vi "slowcont.vi"() -> ()   [LabVIEW 2012]
uses:
  <vilib>/Instr/_visa.llb/VISA Configure Serial Port (Instr).vi
panel:
  out "total magnetic field":dbl(graph)
  out "magnetic field z coordinate":dbl(graph)
  out "magnetic field y coordinate":dbl(graph)
  out "magnetic field x coordinate":dbl(graph)
  out "Pressure":dbl(graph)
  out "humidity":dbl(graph)
  out "Temperature":dbl(graph)
  out "array type (2D Dbl) 2":string[](array[string])
  out "array type (2D Dbl)":string[](array[string])
  out "array 2":string[](array[string])
  out "read buffer":string
  in  "stop":bool
  in  "VISA resource name":refnum<visa-resource-name>="COM5"
  in  "XOFF Character":u8=19 format="%.0x"
  in  "XON Character":u8=17 format="%.0x"
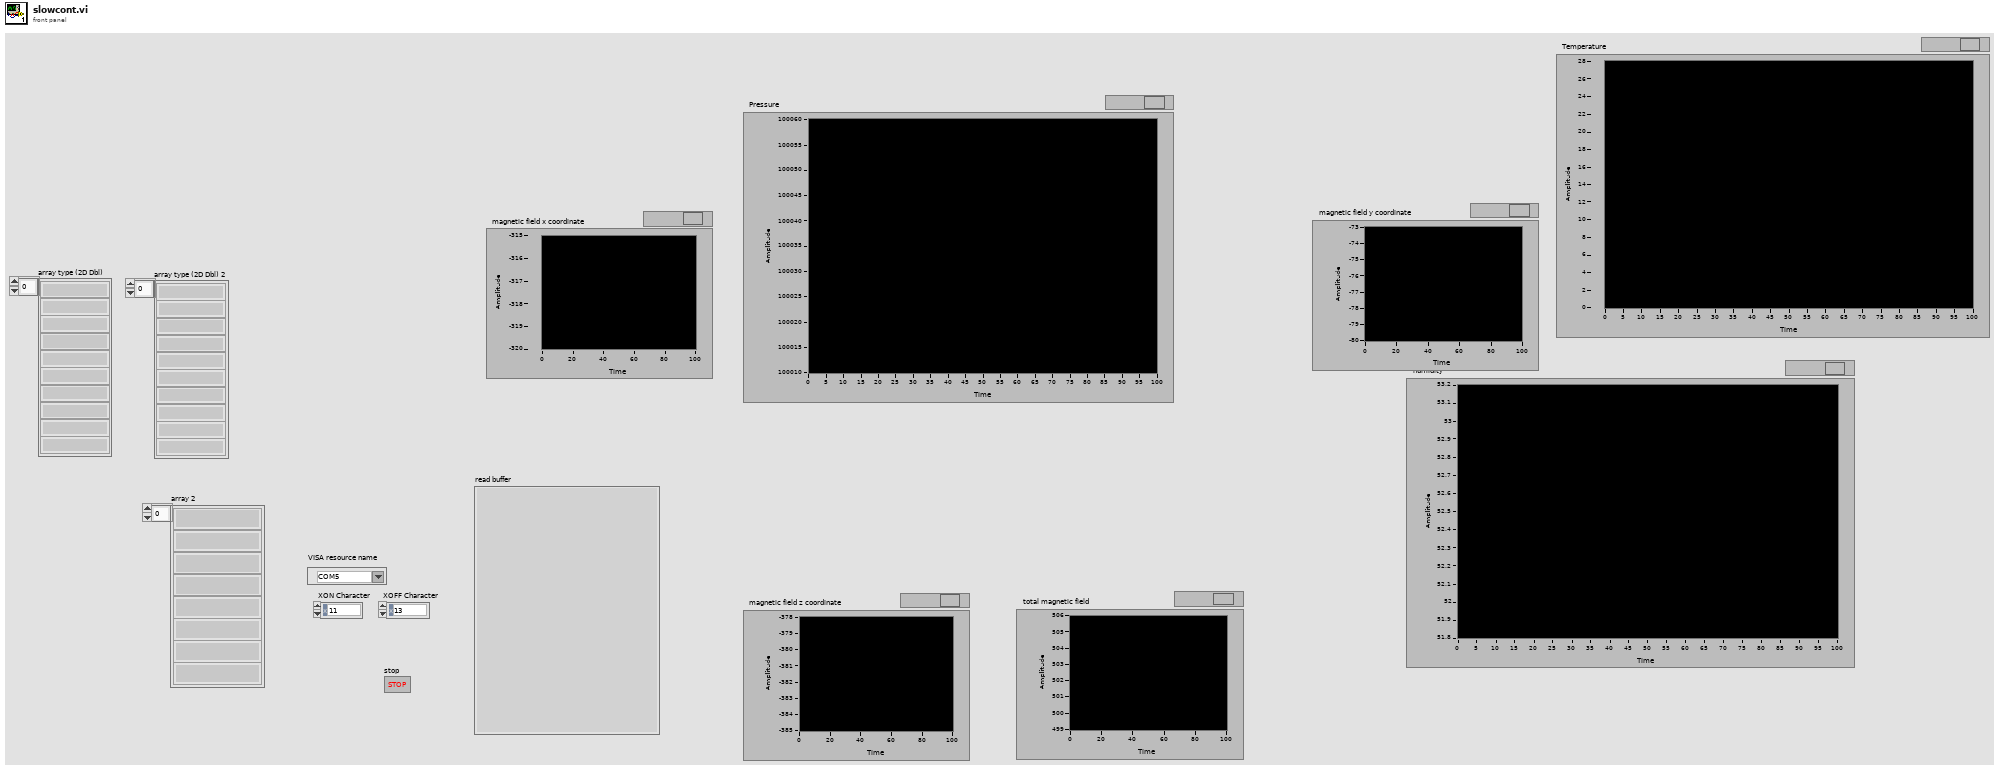
[diagram p1: front panel]
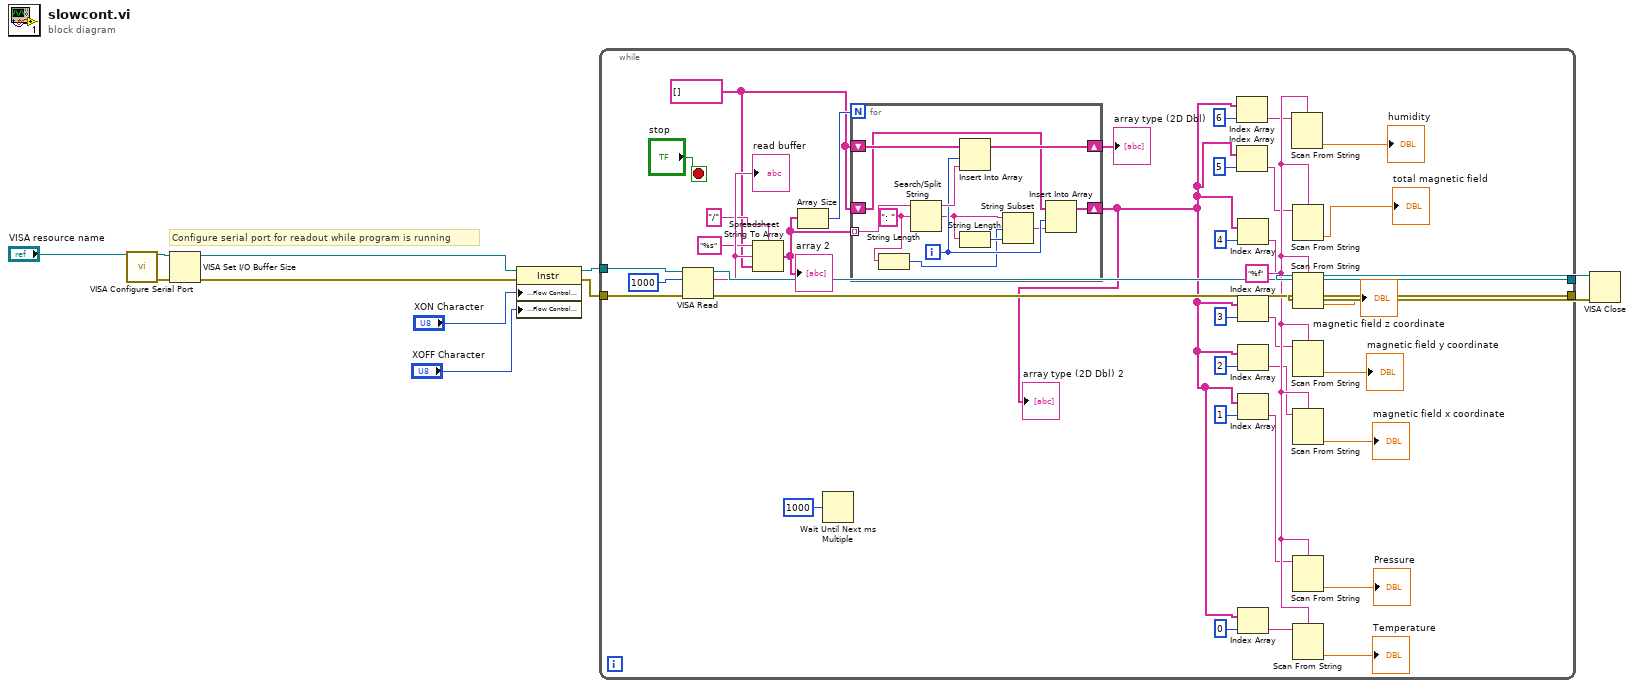
[diagram p0: block diagram]
diagram:
  # "Configure serial port for readout while program is running"
  n1 = call-poly "VISA Configure Serial Port"("VISA resource name"="VISA resource name") -> ("VISA resource name out"=w9:refnum<visa-resource-name>, "error out"=w10:errorcluster)  [unwired: 9 in, 4 out]
  n2 = VISA Set I/O Buffer Size(VISA resource name=w9, error in (no error)=w10) -> (VISA resource name out=w5:refnum<visa-resource-name>, error out=w6:errorcluster)  [unwired: 2 in]
  n3 = property class="Instr"(reference=w5, error in=w6, "Serial Settings:Flow Control XON Character"="XON Character", "Serial Settings:Flow Control XOFF Character"="XOFF Character") -> (reference out=w4:refnum<visa-resource-name>, error out=w3:errorcluster)
  n4 = while {
    tunnel: w4 -> [w46]
    tunnel: w3 -> [w45]
    tunnel: [w44] -> w2
    tunnel: [w43] -> w1
    stop <- "stop" stop-if-true
    w21 = "%f" ("format string")
    w37 = string[] [] ("array type (2D Dbl)")
    n5 = VISA Read(VISA resource name=w46, byte count=u32 1000, error in (no error)=w45) -> (VISA resource name out=w44:refnum<visa-resource-name>, read buffer=w42:string, error out=w43:errorcluster)  [unwired: 1 out]
    "read buffer" <- w42
    n6 = Spreadsheet String To Array(delimiter (Tab)="/", format string="%s", spreadsheet string=w42, array type (2D Dbl)=w37) -> (array=w39:string[])
    "array 2" <- w39
    n7 = Array Size(array=w39) -> (size(s)=w38:i32)
    n8 = Wait Until Next ms Multiple(millisecond multiple=u32 1000) -> ()  [unwired: 1 out]
    n9 = for {
      N: w38 -> [_]
      tunnel: w39 -> [w60] mode=indexing
      shift-right: [w56] -> w36
      shift-left: w37 -> [w59]
      shift-right: [w51] -> w18
      shift-left: w37 -> [w55]
      i -> [w57]
      w50 = ": " ("search string/char (-)")
      n10 = String Length(string=w50) -> (length=w49:i32)
      n11 = Search/Split String(string=w60, search string/char (-)=w50) -> (substring before match=w58:string, match + rest of string=w53:string)  [unwired: 1 in, 1 out]
      n12 = Insert Into Array(array=w59, index=w57, new element=w58) -> (w56:string[])
      n13 = String Length(string=w53) -> (length=w54:i32)
      n14 = String Subset(string=w53, offset (0)=w49, length (rest)=w54) -> (substring=w52:string)
      n15 = Insert Into Array(array=w55, index=w57, new element=w52) -> (w51:string[])
    }
    "array type (2D Dbl)" <- w36
    "array type (2D Dbl) 2" <- w18
    n16 = Index Array(array=w18, index=6) -> (element=w17:string)
    n17 = Index Array(array=w18, index=5) -> (element=w16:string)
    n18 = Index Array(array=w18, index=4) -> (element=w15:string)
    n19 = Index Array(array=w18, index=3) -> (element=w14:string)
    n20 = Index Array(array=w18, index=2) -> (element=w13:string)
    n21 = Index Array(array=w18, index=1) -> (element=w19:string)
    n22 = Index Array(array=w18, index=0) -> (element=w20:string)
    n23 = Scan From String(format string=w21, input string=w17) -> (output 1=→"humidity":dbl)  [unwired: 3 in, 3 out]
    n24 = Scan From String(format string=w21, input string=w16) -> (output 1=→"total magnetic field":dbl)  [unwired: 3 in, 3 out]
    n25 = Scan From String(format string=w21, input string=w15) -> (output 1=→"magnetic field z coordinate":dbl)  [unwired: 3 in, 3 out]
    n26 = Scan From String(format string=w21, input string=w14) -> (output 1=→"magnetic field y coordinate":dbl)  [unwired: 3 in, 3 out]
    n27 = Scan From String(format string=w21, input string=w13) -> (output 1=→"magnetic field x coordinate":dbl)  [unwired: 3 in, 3 out]
    n28 = Scan From String(format string=w21, input string=w19) -> (output 1=→"Pressure":dbl)  [unwired: 3 in, 3 out]
    n29 = Scan From String(format string=w21, input string=w20) -> (output 1=→"Temperature":dbl)  [unwired: 3 in, 3 out]
  }
  n30 = VISA Close(VISA resource name=w2, error in (no error)=w1) -> ()  [unwired: 1 out]
